vi "UV-vis HP 8452A.vi"(4 "function":i32(slide) scale=0.0..3.0, 5 "integration time":ext=0.5 format="%.1f", 6 "stop":ext=820.0, 7 "start":ext=190.0) -> (1 "variance":ext[](array[numeric]) format="%.3e", 2 "measurement":ext[](array[numeric]) format="%.3e")   [LabVIEW 2010]
panel:
  out "Absorption spectrum":cluster{"start":ext, ext, ext[][]}(graph)
  in  "Number of spectra":i32=1
  in  "time between\nmeasurements":u32
  out "error":ext
  # "RUN"
  # "wavelength (nm)"
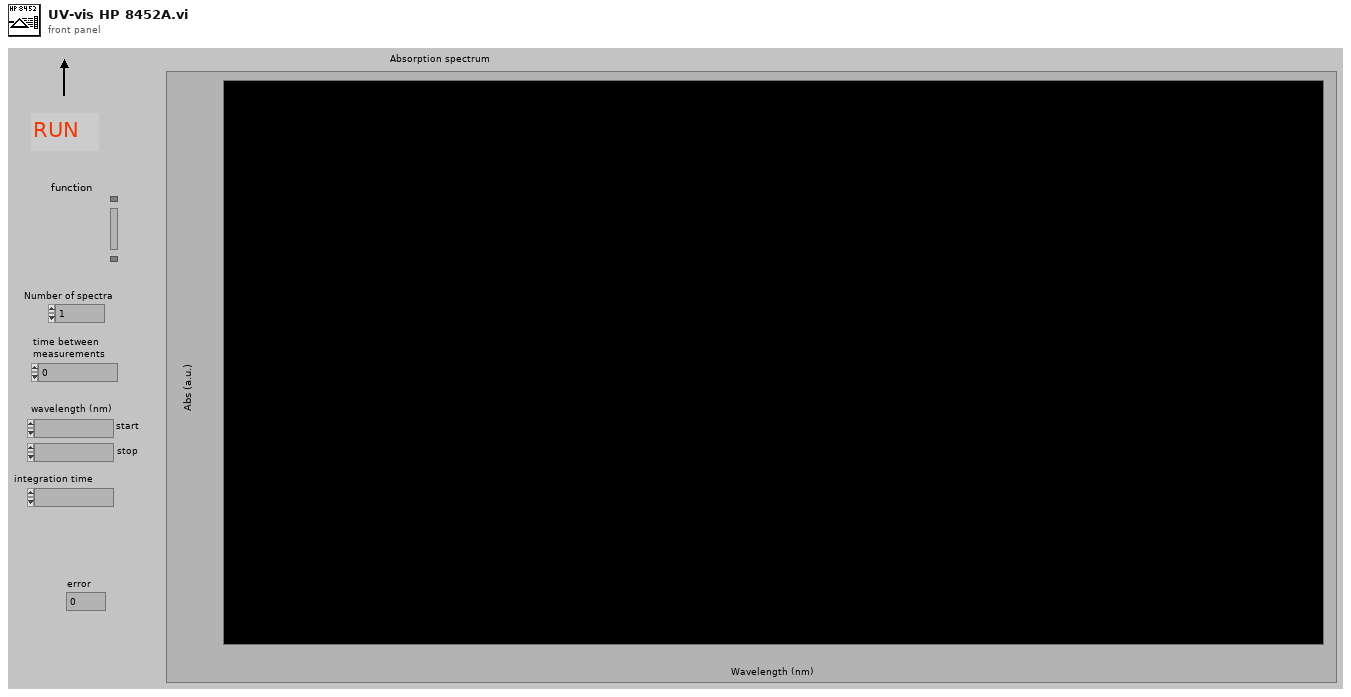
[diagram p1: front panel]
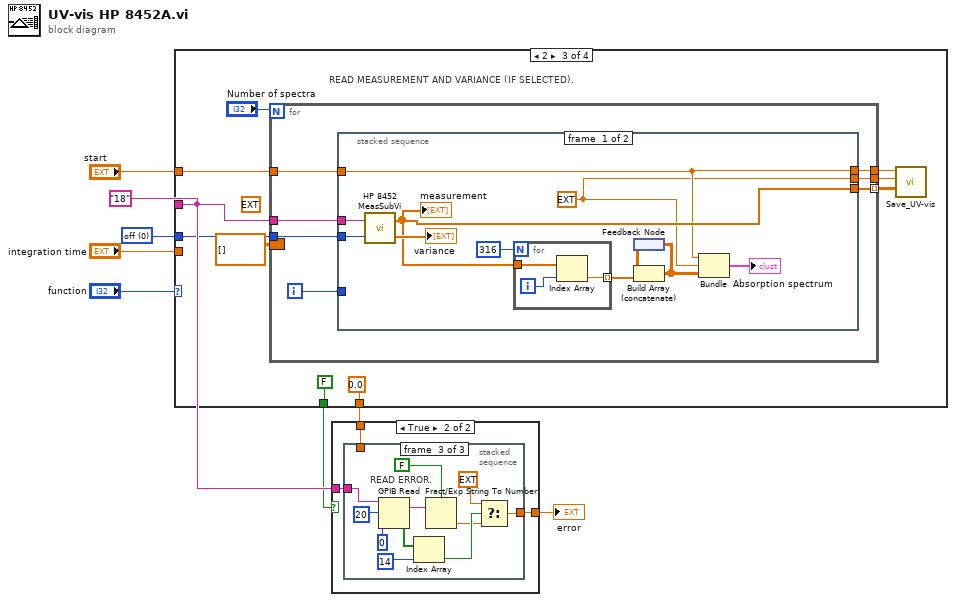
[diagram p0: block diagram]
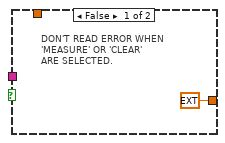
[diagram p2: hidden frame]
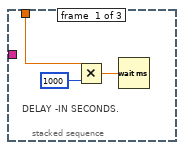
[diagram p3: hidden frame]
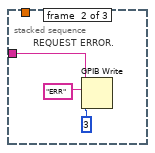
[diagram p4: hidden frame]
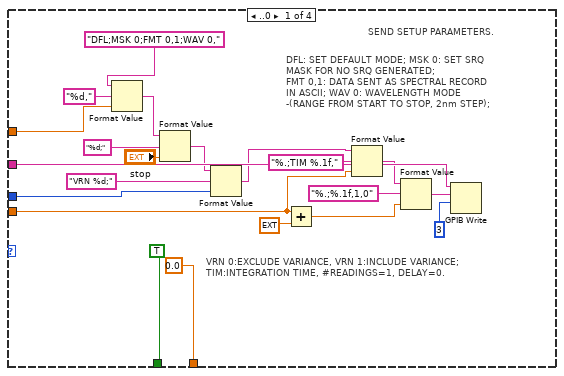
[diagram p5: hidden frame]
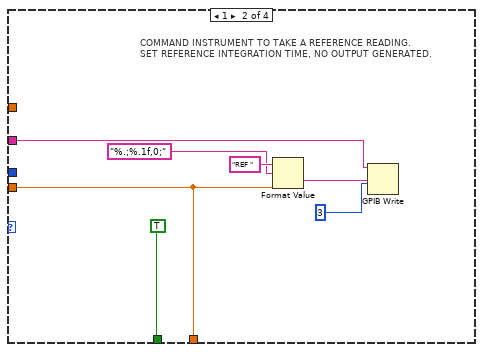
[diagram p6: hidden frame]
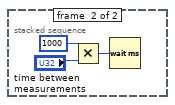
[diagram p7: hidden frame]
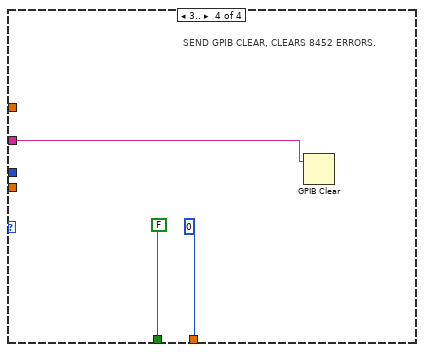
[diagram p8: hidden frame]
diagram:
  w2 = u16 0 items=["off", "on"] ("variance (off:0)")
  w8 = "18"
  n1 = case shown="2" "function" {
    tunnel: "start" -> [w12 _ w42 _]
    tunnel: w2 -> [w17 _ w43 _]
    tunnel: w8 -> [w27 w33 w44 w71]
    tunnel: "integration time" -> [w18 w36 _ _]
    tunnel: [TRUE TRUE FALSE FALSE] -> w5
    tunnel: [0.0 w36 0.0 0] -> w6
    frame ..0 {
      # "DFL: SET DEFAULT MODE; MSK 0: SET SRQ\nMASK FOR NO SRQ GENERATED;\nFMT 0,1: DATA SENT AS SPECTRAL RECORD\nIN ASCII; WAV 0: WAVELENGTH MODE\n-(RANGE FROM START TO STOP, 2nm STEP);"
      # "SEND SETUP PARAMETERS."
      # "VRN 0:EXCLUDE VARIANCE, VRN 1:INCLUDE VARIANCE;\nTIM:INTEGRATION TIME, #READINGS=1, DELAY=0."
      n2 = Format Value(string ("")="DFL;MSK 0;FMT 0,1;WAV 0,", format string="%d,", value (0)=w12) -> (output string=w11:string)
      n3 = Format Value(string ("")=w11, format string="%d;", value (0)="stop") -> (output string=w15:string)
      n4 = Format Value(string ("")=w15, format string="VRN %d;", value (0)=w17) -> (output string=w20:string)
      n5 = Add(x=w18, y=ext 0.5) -> (x+y=w24:ext)
      n6 = Format Value(string ("")=w20, format string="%.;TIM %.1f,", value (0)=w18) -> (output string=w22:string)
      n7 = Format Value(string ("")=w22, format string="%.;%.1f,1,0", value (0)=w24) -> (output string=w25:string)
      n8 = GPIB Write(0:w27, 1:w25, 2:3) -> ()  [unwired: 2 in, 2 out]
    }
    frame 1 {
      # "COMMAND INSTRUMENT TO TAKE A REFERENCE READING.\nSET REFERENCE INTEGRATION TIME, NO OUTPUT GENERATED."
      n9 = Format Value(string ("")="REF ", format string="%.;%.1f,0;", value (0)=w36) -> (output string=w30:string)
      n10 = GPIB Write(0:w33, 1:w30, 2:3) -> ()  [unwired: 2 in, 2 out]
    }
    frame 2 {
      (unwired) ext 0.0
      # "READ MEASUREMENT AND VARIANCE (IF SELECTED)."
      n11 = for {
        N: "Number of spectra" -> [_]
        tunnel: w44 -> [w53]
        tunnel: w43 -> [w52]
        tunnel: w42 -> [w51]
        tunnel: [w50] -> w40
        tunnel: [w49] -> w39
        tunnel: [w48] -> w38 mode=indexing
        border: ext[][] [] -> [_]
        i -> [w47]
        n12 = stacked-sequence {
          tunnel: w53 -> [w64 _]
          tunnel: w52 -> [w62 _]
          tunnel: w51 -> [w57 _]
          tunnel: [w57 _] -> w50
          tunnel: [w56 _] -> w49
          tunnel: [w60 _] -> w48
          tunnel: w47 -> [_ _]
          frame #0 {
            w56 = ext 2.0
            n13 = call <instrlib>:"HP 8452 MeasSubVi.vi"("variance option (off:0)"=w62, "GPIB"=w64) -> ("variance"=→"variance":ext[], "measurement"=w60:ext[])
            "measurement" <- w60
            n14 = for {
              N: 316 -> [_]
              tunnel: w60 -> [w67]
              tunnel: [w65] -> w59 mode=indexing
              i -> [w66]
              n15 = Index Array(array=w67, index=w66) -> (element=w65:ext)
            }
            n16 = feedback #1() -> (w58:ext[][])
            n17 = Build Array (concatenate)(w58, w59) -> (w55:ext[][])
            n18 = feedback-in #1(w55) -> ()
            n19 = Bundle("start"=w57, w56, w55) -> (→"Absorption spectrum":cluster{"start":ext, ext, ext[][]})  [unwired: 1 in]
          }
          frame #1 {
            n20 = Multiply(x=1000, y="time between\nmeasurements") -> (x*y=w68:u32)
            n21 = Wait (ms)(milliseconds to wait=w68) -> ()  [unwired: 1 out]
          }
        }
      }
      n22 = call <userlib>:"Save_UV-vis.vi"("measurement"=w38, "step"=w39, "start"=w40) -> ()  [unwired: 8 in, 1 out]
    }
    frame 3.. {
      # "SEND GPIB CLEAR, CLEARS 8452 ERRORS."
      n23 = GPIB Clear(3:w71) -> ()  [unwired: 1 in, 2 out]
    }
  }
  n24 = case shown="True" w5 {
    tunnel: w6 -> [_ w75]
    tunnel: [ext 0.0 w76] -> w7
    tunnel: w8 -> [_ w77]
    frame False {
      # "DON'T READ ERROR WHEN\n'MEASURE' OR 'CLEAR'\nARE SELECTED."
    }
    frame True {
      n25 = stacked-sequence {
        tunnel: w75 -> [w78 _ _]
        tunnel: [_ _ w93] -> w76
        tunnel: w77 -> [_ w81 w94]
        frame #0 {
          # "DELAY -IN SECONDS."
          n26 = Multiply(x=w78, y=1000) -> (x*y=w80:ext)
          n27 = Wait (ms)(milliseconds to wait=w80) -> ()  [unwired: 1 out]
        }
        frame #1 {
          # "REQUEST ERROR."
          n28 = GPIB Write(0:w81, 1:"ERR", 2:3) -> ()  [unwired: 2 in, 2 out]
        }
        frame #2 {
          # "READ ERROR."
          n29 = GPIB Read(0:w94, 1:20, 2:0) -> (5:w87:string, 6:w88:bool[])  [unwired: 2 in, 1 out]
          n30 = Index Array(array=w88, index=14) -> (element=w91:bool)
          n31 = Fract/Exp String To Number(use system decimal point (T)=FALSE, string=w87) -> (number=w90:dbl)  [unwired: 2 in, 1 out]
          n32 = Select(t=ext -1.0, s=w91, f=w90) -> (s? t:f=w93:ext)
        }
      }
    }
  }
  "error" <- w7
